vi "load methods.vi"(8 "error in (no error)":errorcluster, 10 "Folder Path":path) -> (0 "error out":errorcluster, 3 "Method Manager out":refnum<class "Method Loader.lvclass">)   [LabVIEW 2020, in "JSON-RPC Lib.lvlib" / "Method Loader.lvclass"]
uses:
  Method Loader.lvclass
  method type.ctl
  Method Loader.lvclass/Method Loader.ctl
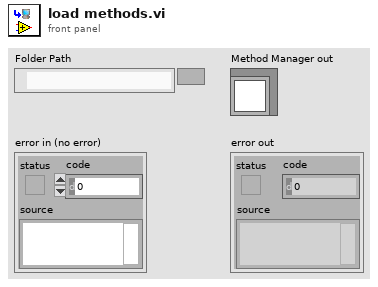
[diagram p1: front panel]
types:
  T1 = typedef "JSON-RPC Lib.lvlib/Method Loader.lvclass/method type.ctl" = refnum<vi>
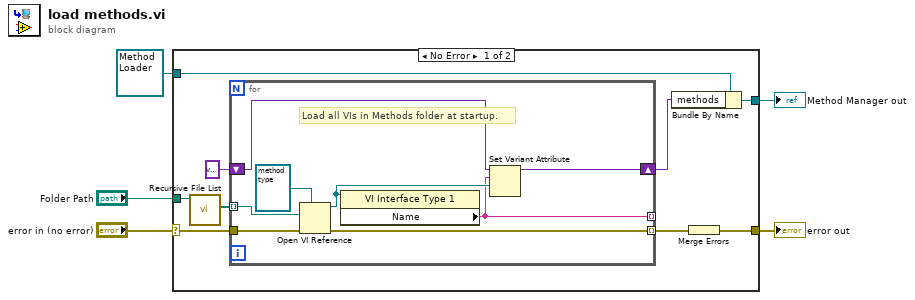
[diagram p0: block diagram]
diagram:
  n1 = case shown="No Error" "error in (no error)" {
    selector: "error in (no error)" -> [w9 w24]
    tunnel: [w12 w24] -> w3
    tunnel: "Folder Path" -> [w11 _]
    tunnel: refnum<class "Method Loader.lvclass"> refnum ("Method Manager in") -> [w8 w23]
    tunnel: [w6 w23] -> w1
    frame No Error {
      n2 = call <vilib>:"Recursive File List.vi"("Folder Path"=w11) -> ("All Files in Dir"=w10:path[])  [unwired: 6 in, 4 out]
      n3 = for {
        tunnel: w10 -> [w22] mode=indexing
        tunnel: [w21] -> w13 mode=indexing
        shift-right: [w20] -> w7
        shift-left: variant -> [w19]
        tunnel: [w17] -> _ mode=indexing
        tunnel: w9 -> [w15]
        # "Load all VIs in Methods folder at startup."
        n4 = Open VI Reference(type specifier VI Refnum (for type only)=T1 refnum, vi path=w22, error in (no error)=w15) -> (vi reference=w18:T1, error out=w21:errorcluster)  [unwired: 3 in]
        n5 = property class="VI Interface Type 1"(reference=w18) -> ("Name"=w17:string)  [unwired: 1 in, 2 out]
        n6 = Set Variant Attribute(Variant=w19, name=w17, value=w18) -> (Variant out=w20:variant)  [unwired: 1 in, 2 out]
      }
      n7 = Bundle By Name(cluster=w8, "methods"=w7) -> (w6:refnum<class "Method Loader.lvclass">)
      n8 = Merge Errors(w13) -> (w12:errorcluster)
    }
    frame Error {
    }
  }
  "error out" <- w3
  "Method Manager out" <- w1
